vi "Calibrate Polarizer.vi"(8 "error in (no error)":errorcluster, 11 "Laser in":refnum<class "Laser.lvclass">) -> (0 "error out":errorcluster, 2 "best fit parameters":dbl[](array[numeric]), 3 "Laser out":refnum<class "Laser.lvclass">, 9 "Angle (deg)":dbl[](array[numeric]), 10 "Power (W)":dbl[](array[numeric]))   [LabVIEW 2018, in "Laser.lvlib" / "Laser.lvclass"]
uses:
  Laser.lvclass
  Laser.lvclass/Laser.ctl
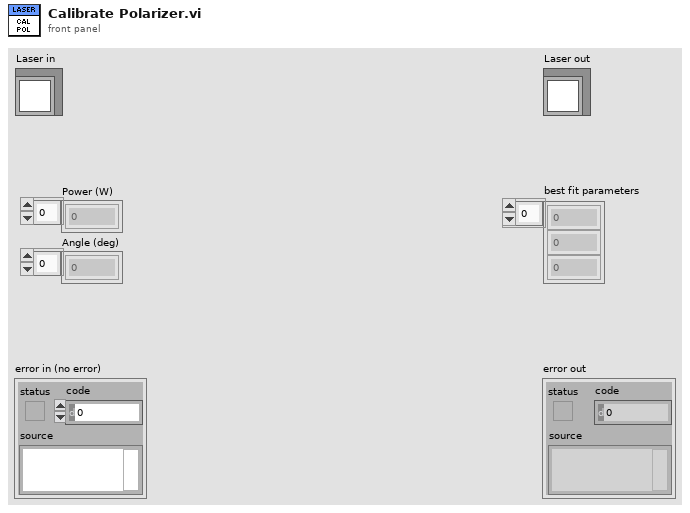
[diagram p1: front panel]
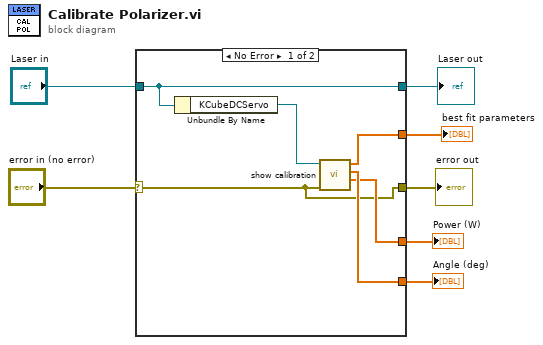
[diagram p0: block diagram]
diagram:
  n1 = case shown="No Error" "error in (no error)" {
    selector: "error in (no error)" -> [w8 w15]
    tunnel: [w8 w15] -> w6
    tunnel: [w13 w14] -> w4
    tunnel: "Laser in" -> [w13 w14]
    tunnel: [w9 _] -> w3
    tunnel: [w10 _] -> w2
    tunnel: [w11 _] -> w1
    frame No Error {
      n2 = Unbundle By Name(w13) -> ("KCubeDCServo"=w12:refnum<k24>)
      n3 = call "show calibration.vi"("error in"=w8, "KCubeDCServo"=w12) -> ("Power (W)"=w9:dbl[], "Angle (degrees)"=w10:dbl[], "best fit parameters"=w11:dbl[])  [unwired: 4 in, 1 out]
    }
    frame Error {
    }
  }
  "error out" <- w6
  "Laser out" <- w4
  "Power (W)" <- w3
  "Angle (deg)" <- w2
  "best fit parameters" <- w1
